vi "ClearBits(U16).vi"(8 "error in (no error)":errorcluster caption="错误输入（无错误）", 10 "Clear":bool=TRUE, 11 "Input(U16)":u16 format="%.0x") -> (0 "error out":errorcluster caption="错误输出", 3 "Output(U16)":u16 format="%.0x")   [LabVIEW 2012]
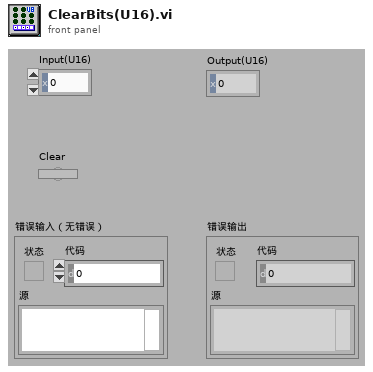
[diagram p1: front panel]
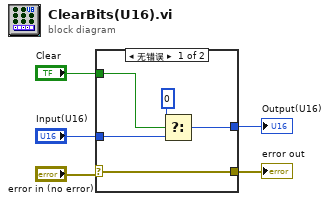
[diagram p0: block diagram]
diagram:
  n1 = case shown="无错误" "error in (no error)" {
    selector: "error in (no error)" -> [w10 w12]
    tunnel: [w10 w12] -> w4
    tunnel: "Input(U16)" -> [w7 w11]
    tunnel: "Clear" -> [w9 _]
    tunnel: [w6 w11] -> w1
    frame No Error {
      n2 = Select(t=u16 0, s=w9, f=w7) -> (s? t:f=w6:u16)
    }
    frame Error {
    }
  }
  "error out" <- w4
  "Output(U16)" <- w1
